vi "visn_Calculate CRC-5 (Bits Array).vi"(11 "Bits Array":u8[](array[numeric])=[1, 1, 0, 0, 1, 1, 1, 0, 1, 0] format="%0x") -> (3 "CRC-5":u8[](array[numeric])=[1, 1, 0, 0, 1] format="%0x")   [LabVIEW 2015]
panel:
  out "loop":i32
  in  "Case Constant\n(See Context Help)":bool
  out "unsigned 32bit integer":u32 format="%b"
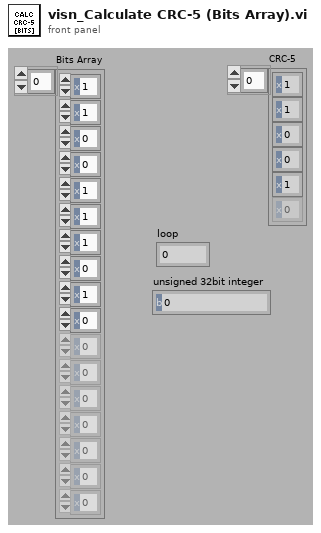
[diagram p1: front panel]
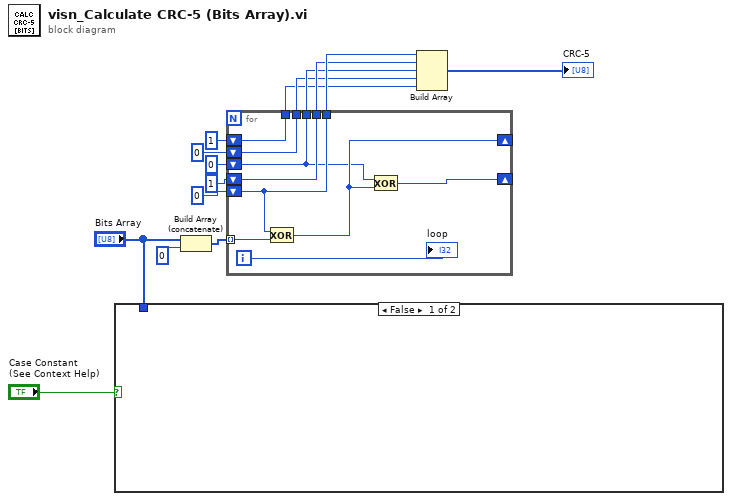
[diagram p0: block diagram]
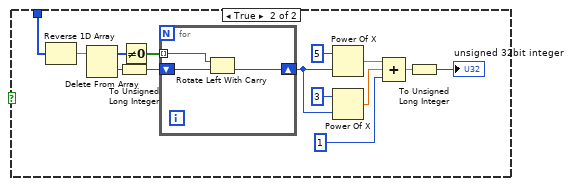
[diagram p2: hidden frame]
diagram:
  n1 = case shown="False" "Case Constant\n(See Context Help)" {
    tunnel: "Bits Array" -> [_ w29]
    frame False {
    }
    frame True {
      n2 = Reverse 1D Array(array=w29) -> (reversed array=w28:u8[])
      n3 = Delete From Array(array=w28) -> (deleted portion=w27:u8, array with subset deleted=w26:u8[])  [unwired: 2 in]
      n4 = To Unsigned Long Integer(number=w27) -> (unsigned 32bit integer=w24:u32)
      n5 = Not Equal To 0?(x=w26) -> (x != 0?=w25:bool[])
      n6 = for {
        shift-right: [w31] -> w22
        shift-left: w24 -> [w32]
        tunnel: w25 -> [w30] mode=indexing
        n7 = Rotate Left With Carry(2:w32, 3:w30) -> (0:w31:u32)  [unwired: 1 out]
      }
      n8 = Power Of X(1:w22, 2:u32 5 ("y")) -> (0:w20:dbl)
      n9 = Power Of X(1:w22, 2:u32 3 ("y")) -> (0:w19:dbl)
      n10 = Compound Arithmetic op=ADD(w20, w19, u32 1 ("y")) -> (w17:dbl)
      n11 = To Unsigned Long Integer(number=w17) -> (unsigned 32bit integer=→"unsigned 32bit integer":u32)
    }
  }
  n12 = Build Array (concatenate)("Bits Array", u8 0) -> (w4:u8[])
  n13 = for {
    shift-right: [w40] -> _
    shift-left: u8 0 -> [w35]
    shift-left: u8 0 -> [w36]
    tunnel: w4 -> [w41] mode=indexing
    shift-right: [w39] -> _
    shift-left: u8 0 -> [w38]
    shift-left: u8 1 -> [w34]
    shift-left: u8 1 -> [w37]
    tunnel: [w38] -> w10
    tunnel: [w37] -> w9
    tunnel: [w36] -> w8
    tunnel: [w35] -> w7
    tunnel: [w34] -> w6
    i -> [w33]
    n14 = Exclusive Or(1:w41, 2:w38) -> (0:w40:u8)
    n15 = Exclusive Or(1:w40, 2:w36) -> (0:w39:u8)
    "loop" <- w33
  }
  n16 = Build Array(w10, w9, w8, w7, w6) -> (→"CRC-5":u8[])
